vi "报警处理.vi"(8 "错误常量":errorcluster caption="错误输入") -> (0 "错误输出":errorcluster, 3 "按钮输出":i32(ring) items=["None", "OK", "Cancel", "Abort", "Retry", "Ignore", "Yes", "No"])   [LabVIEW 2020]
uses:
  <vilib>/Utility/error.llb/DialogType.ctl
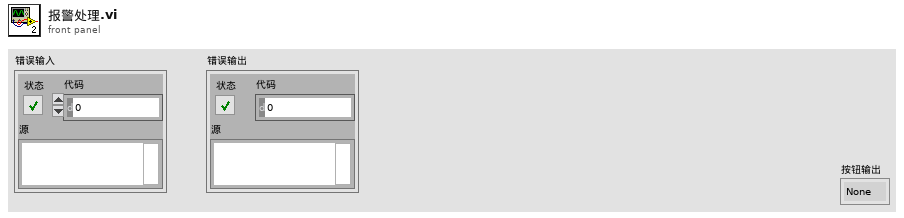
[diagram p1: front panel]
types:
  T1 = typedef "DialogType.ctl" = u16
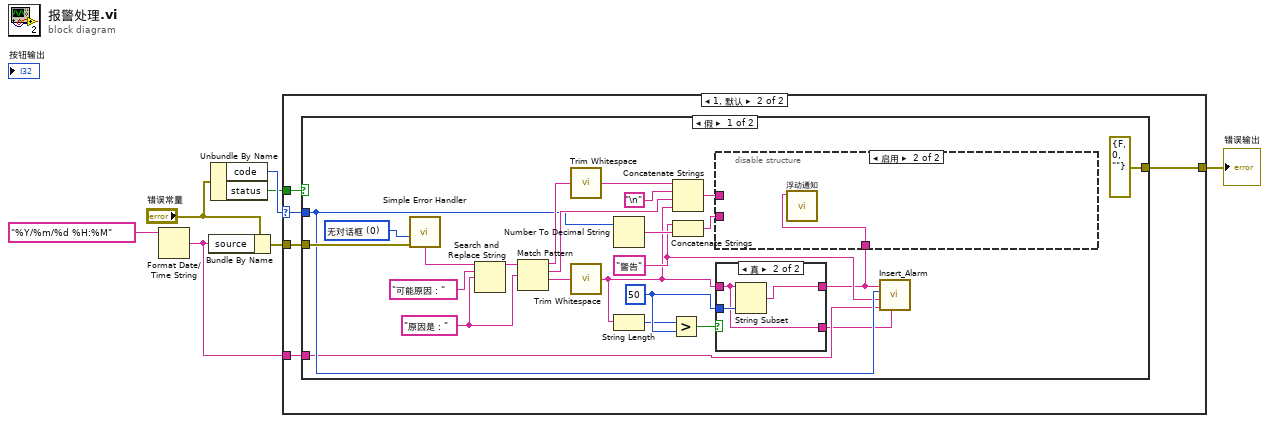
[diagram p0: block diagram]
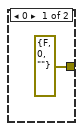
[diagram p2: hidden frame]
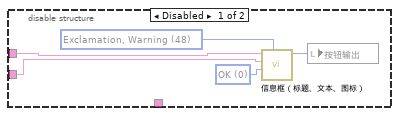
[diagram p3: hidden frame]
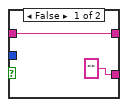
[diagram p4: hidden frame]
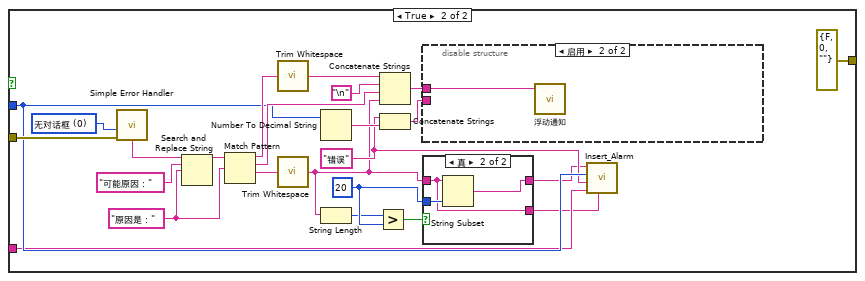
[diagram p5: hidden frame]
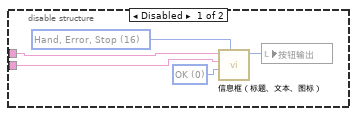
[diagram p6: hidden frame]
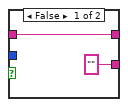
[diagram p7: hidden frame]
diagram:
  n1 = Format Date/Time String(time format string (%c)="%Y/%m/%d %H:%M" ("时间格式字符串(%c)")) -> (date/time string=w6:string)  [unwired: 2 in]
  n2 = Bundle By Name(cluster="错误常量", "source"=w6) -> (w4:errorcluster)
  n3 = Unbundle By Name("错误常量") -> ("code"=w3:i32, "status"=w1:bool)
  n4 = case shown="1, 默认" w3 {
    selector: w3 -> [_ w12]
    tunnel: w4 -> [_ w13]
    tunnel: w6 -> [_ w11]
    tunnel: [errorcluster {"status"=FALSE, "code"=0, "source"=""} ("错误输出") w10] -> w5
    tunnel: w1 -> [_ w9]
    frame 0 {
    }
    frame 1, Default {
      n5 = case shown="假" w9 {
        tunnel: w13 -> [w37 w72]
        tunnel: w12 -> [w25 w59]
        tunnel: w11 -> [w24 w58]
        tunnel: [errorcluster {"status"=FALSE, "code"=0, "source"=""} ("错误输出") errorcluster {"status"=FALSE, "code"=0, "source"=""} ("错误输出")] -> w10
        frame False {
          w21 = 50 ("y")
          w16 = "原因是：" ("字符串")
          w29 = T1 0 items=["无对话框", "确定信息", "继续或停止信息", "确定信息＋警告", "继续/停止+警告"] ("type of dialog (OK msg:1)")
          w23 = "警告" ("caption")
          n6 = call <vilib>:"Simple Error Handler.vi"("type of dialog (OK msg:1)"=w29, "error in (no error)"=w37) -> ("message"=w28:string)  [unwired: 3 in, 4 out]
          n7 = Search and Replace String(input string=w28, search string="可能原因：" ("正则表达式"), replace string=w16) -> (result string=w15:string)  [unwired: 5 in, 3 out]
          n8 = Match Pattern(string=w15, regular expression=w16) -> (before substring=w33:string, match substring=w26:string, after substring=w36:string)  [unwired: 1 in, 1 out]
          n9 = call <vilib>:"Trim Whitespace.vi"("string"=w33) -> ("trimmed string"=w32:string)  [unwired: 1 in]
          n10 = call <vilib>:"Trim Whitespace.vi"("string"=w36) -> ("trimmed string"=w18:string)  [unwired: 1 in]
          n11 = Number To Decimal String(number=w25) -> (decimal integer string=w31:string)  [unwired: 1 in]
          n12 = String Length(string=w18) -> (length=w19:i32)
          n13 = Greater?(x=w19, y=w21) -> (0:w20:bool)
          n14 = Concatenate Strings(w32, "\n", w26, w18) -> (w34:string)
          n15 = Concatenate Strings(w23, w31) -> (w30:string)
          n16 = case shown="真" w20 {
            tunnel: w18 -> [w44 w46]
            tunnel: w21 -> [_ w48]
            tunnel: [w44 w47] -> w14
            tunnel: ["" ("trimmed string") w46] -> w17
            frame False {
            }
            frame True {
              n17 = String Subset(string=w46, length (rest)=w48) -> (substring=w47:string)  [unwired: 1 in]
            }
          }
          n18 = disable-structure shown="启用" {
            disable-tunnel: w34 -> [w42 _]
            disable-tunnel: w30 -> [w39 _]
            disable-tunnel: w14 -> [_ w43]
            frame Disabled {
              w40 = 0 items=["OK", "OKCancel", "AbortRetryIgnore", "YesNoCancel", "YesNo", "RetryCancel"] ("buttons")
              w41 = 48 items=["None"=0, "Hand, Error, Stop"=16, "Question"=32, "Exclamation, Warning"=48, "Asterisk, Information"=64] ("icon")
              n19 = call "信息框（标题、文本、图标）.vi"("icon"=w41, "buttons"=w40, "caption"=w39, "text"=w42) -> ("按钮输出"=w38:i32)  [unwired: 6 in, 1 out]
              n20 = local write "按钮输出"(w38) -> ()
            }
            frame Enabled {
              n21 = call "浮动通知.vi"("通知内容"=w43) -> ()  [unwired: 11 in]
            }
          }
          n22 = call "Insert_Alarm.vi"("备注"=w17, "报警时间"=w24, "报警类型"=w23, "报警代码"=w25, "报警名称"=w14) -> ()  [unwired: 1 in, 1 out]
        }
        frame True {
          w54 = 20 ("y")
          w61 = "原因是：" ("字符串")
          w65 = T1 0 items=["无对话框", "确定信息", "继续或停止信息", "确定信息＋警告", "继续/停止+警告"] ("type of dialog (OK msg:1)")
          w56 = "错误" ("caption")
          n23 = call <vilib>:"Simple Error Handler.vi"("type of dialog (OK msg:1)"=w65, "error in (no error)"=w72) -> ("message"=w63:string)  [unwired: 3 in, 4 out]
          n24 = Search and Replace String(input string=w63, search string="可能原因：" ("正则表达式"), replace string=w61) -> (result string=w64:string)  [unwired: 5 in, 3 out]
          n25 = Match Pattern(string=w64, regular expression=w61) -> (before substring=w69:string, match substring=w60:string, after substring=w71:string)  [unwired: 1 in, 1 out]
          n26 = call <vilib>:"Trim Whitespace.vi"("string"=w69) -> ("trimmed string"=w68:string)  [unwired: 1 in]
          n27 = call <vilib>:"Trim Whitespace.vi"("string"=w71) -> ("trimmed string"=w51:string)  [unwired: 1 in]
          n28 = Number To Decimal String(number=w59) -> (decimal integer string=w67:string)  [unwired: 1 in]
          n29 = String Length(string=w51) -> (length=w52:i32)
          n30 = Greater?(x=w52, y=w54) -> (0:w53:bool)
          n31 = Concatenate Strings(w68, "\n", w60, w51) -> (w57:string)
          n32 = Concatenate Strings(w56, w67) -> (w66:string)
          n33 = disable-structure shown="启用" {
            disable-tunnel: w66 -> [w75 _]
            disable-tunnel: w57 -> [w74 w78]
            frame Disabled {
              w76 = 0 items=["OK", "OKCancel", "AbortRetryIgnore", "YesNoCancel", "YesNo", "RetryCancel"] ("buttons")
              w77 = 16 items=["None"=0, "Hand, Error, Stop"=16, "Question"=32, "Exclamation, Warning"=48, "Asterisk, Information"=64] ("icon")
              n34 = call "信息框（标题、文本、图标）.vi"("icon"=w77, "buttons"=w76, "caption"=w75, "text"=w74) -> ("按钮输出"=w73:i32)  [unwired: 6 in, 1 out]
              n35 = local write "按钮输出"(w73) -> ()
            }
            frame Enabled {
              n36 = call "浮动通知.vi"("通知内容"=w78) -> ()  [unwired: 11 in]
            }
          }
          n37 = case shown="真" w53 {
            tunnel: w51 -> [w79 w81]
            tunnel: w54 -> [_ w83]
            tunnel: [w79 w82] -> w50
            tunnel: ["" ("trimmed string") w81] -> w49
            frame False {
            }
            frame True {
              n38 = String Subset(string=w81, length (rest)=w83) -> (substring=w82:string)  [unwired: 1 in]
            }
          }
          n39 = call "Insert_Alarm.vi"("备注"=w49, "报警时间"=w58, "报警类型"=w56, "报警代码"=w59, "报警名称"=w50) -> ()  [unwired: 1 in, 1 out]
        }
      }
    }
  }
  "错误输出" <- w5
